vi "Write to DB_12202024.vi"(8 "error in (no error)":errorcluster, 11 "Database Entry in":refnum<class "Database Entry.lvclass">) -> (0 "error out":errorcluster, 2 "Stack names":string[](array[string]), 3 "Database Entry out":refnum<class "Database Entry.lvclass">)   [LabVIEW 2021, in "Database Entry.lvclass"]
uses:
  Database Entry.lvclass
  Database Entry.lvclass/Database Entry.ctl
  <vilib>/Utility/file.llb/Read Delimited Spreadsheet (string).vi
  <vilib>/Utility/file.llb/Write Delimited Spreadsheet (string).vi
  Components/Stack/Stack.lvclass
panel:
  out "Final name":string
  out "Data cluster":T1={"module or proto"="proto", " geometry"="full", "resolution"="LD", "baselayer"="BA_123", "toplayer"="SI_789", "bl_pos"="1", "tl_pos"="1", "put_pos"="1", "region"="1", "asstray"="1", "comptray"="1", "put"="1", "date"="2024-04-02", "timestart"="1:12:12.442", "timeend"="1:23:45.244", "operator"="cmuperson", "tape"="some", "glue"="some", "stack name"="some", "Adhesive type"="", "Comments"="", "Temperature"="", "Relative Humidity"=""}
  out "error out py":errorcluster
  out "String Out":string="Upload Success"
  in  "error in (no error) py":errorcluster
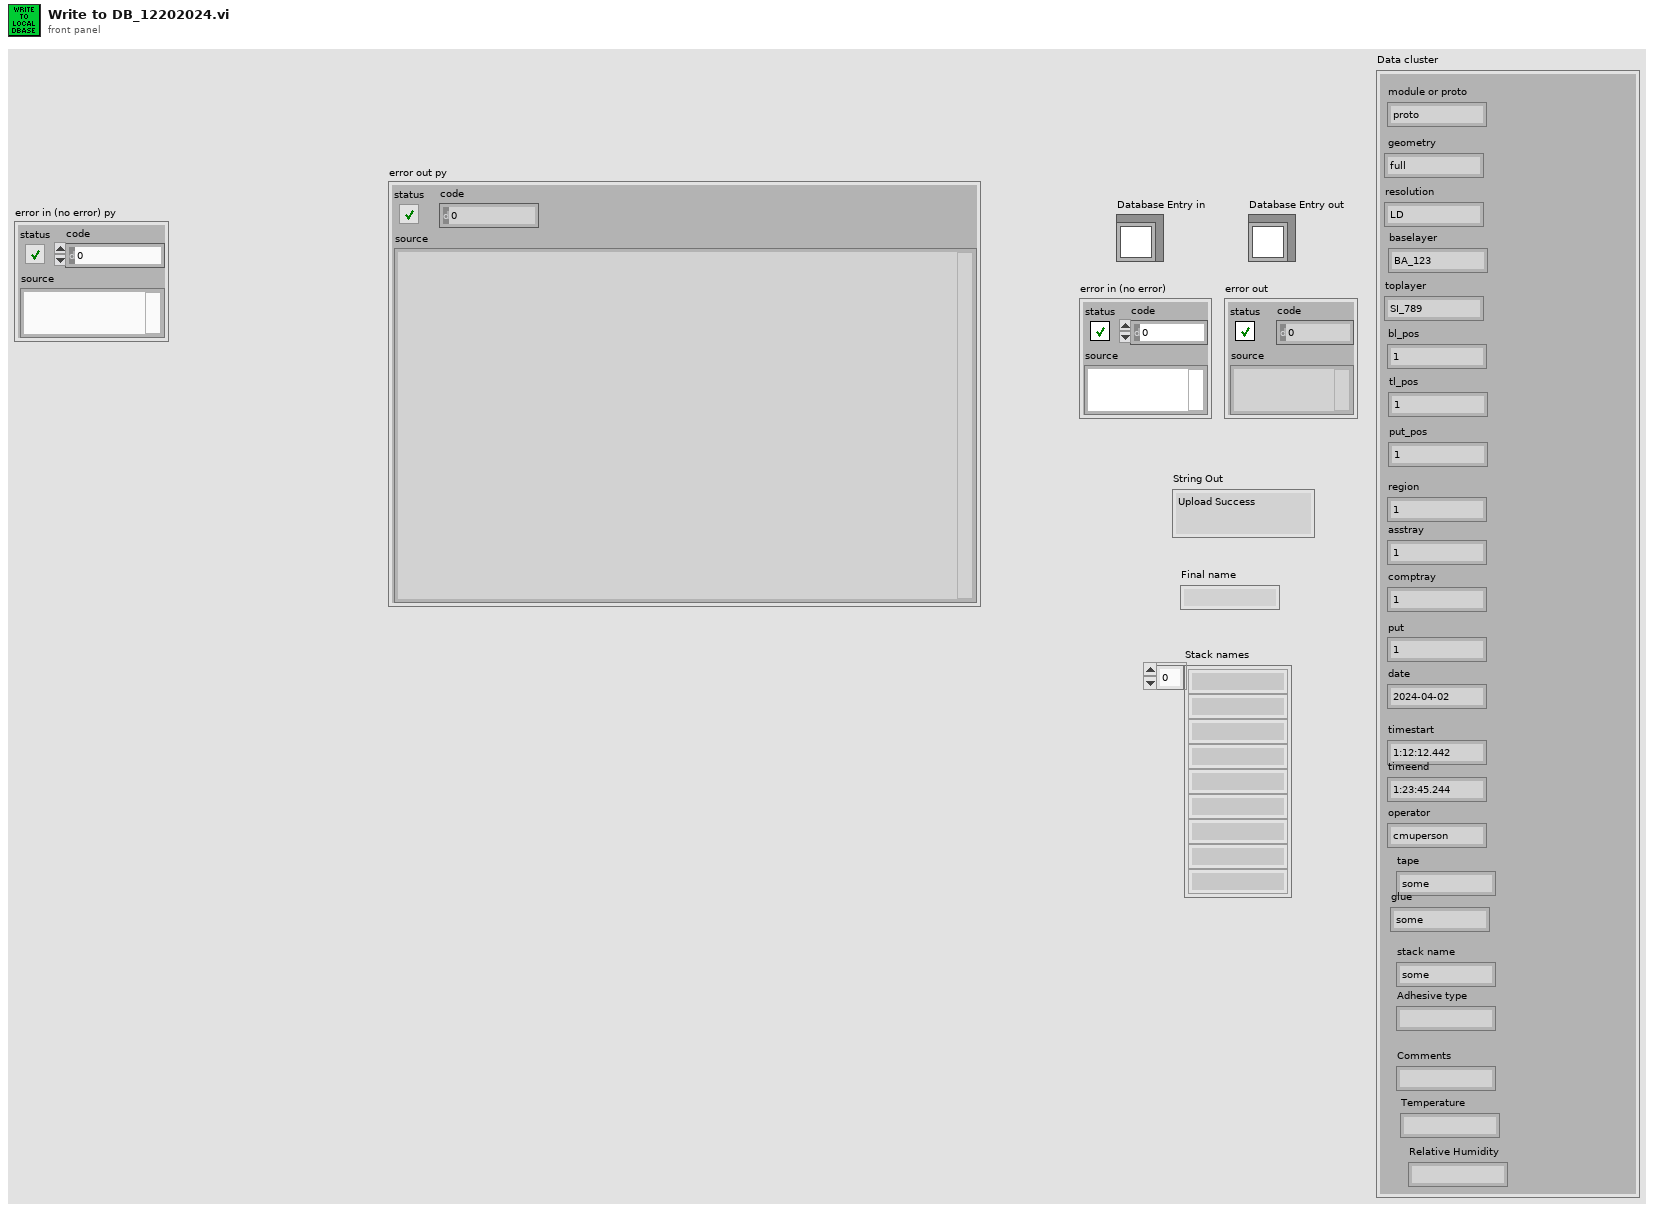
[diagram p1: front panel]
types:
  T1 = cluster{"module or proto":string, " geometry":string, "resolution":string, "baselayer":string, "toplayer":string, "bl_pos":string, "tl_pos":string, "put_pos":string, "region":string, "asstray":string, "comptray":string, "put":string, "date":string, "timestart":string, "timeend":string, "operator":string, "tape":string, "glue":string, "stack name":string, "Adhesive type":string, "Comments":string, "Temperature":string, "Relative Humidity":string}
  T2 = typedef "File Paths.ctl" = cluster{"Glue Pattern Folder":path, "Carrier Tray Folder":path, "Pick Up Tool Fixture Folder":path, "Components Folder":path, "Bellows Tool Offset.txt":path, "Pick Up Tool Offset.txt":path, "Dispense Tip Offset.txt":path, "Log Files":path, "Gantry Assembly Map.txt":path, "Syringe and offset map.txt":path, "Controllers Folder":path, "Local dbase config":path}
  T3 = cluster{"type":string, " geometry":string, "resolution":string, "baselayer":string, "toplayer":string, "bl_pos":string, "tl_pos":string, "put_pos":string, "region":string, "asstray":string, "comptray":string, "put":string, "date":string, "timestart":string, "timeend":string, "operator":string, "tape":string, "glue":string, "stack name":string, "Adhesive type":string, "Comments":string, "Temperature":string, "Relative Humidity":string}
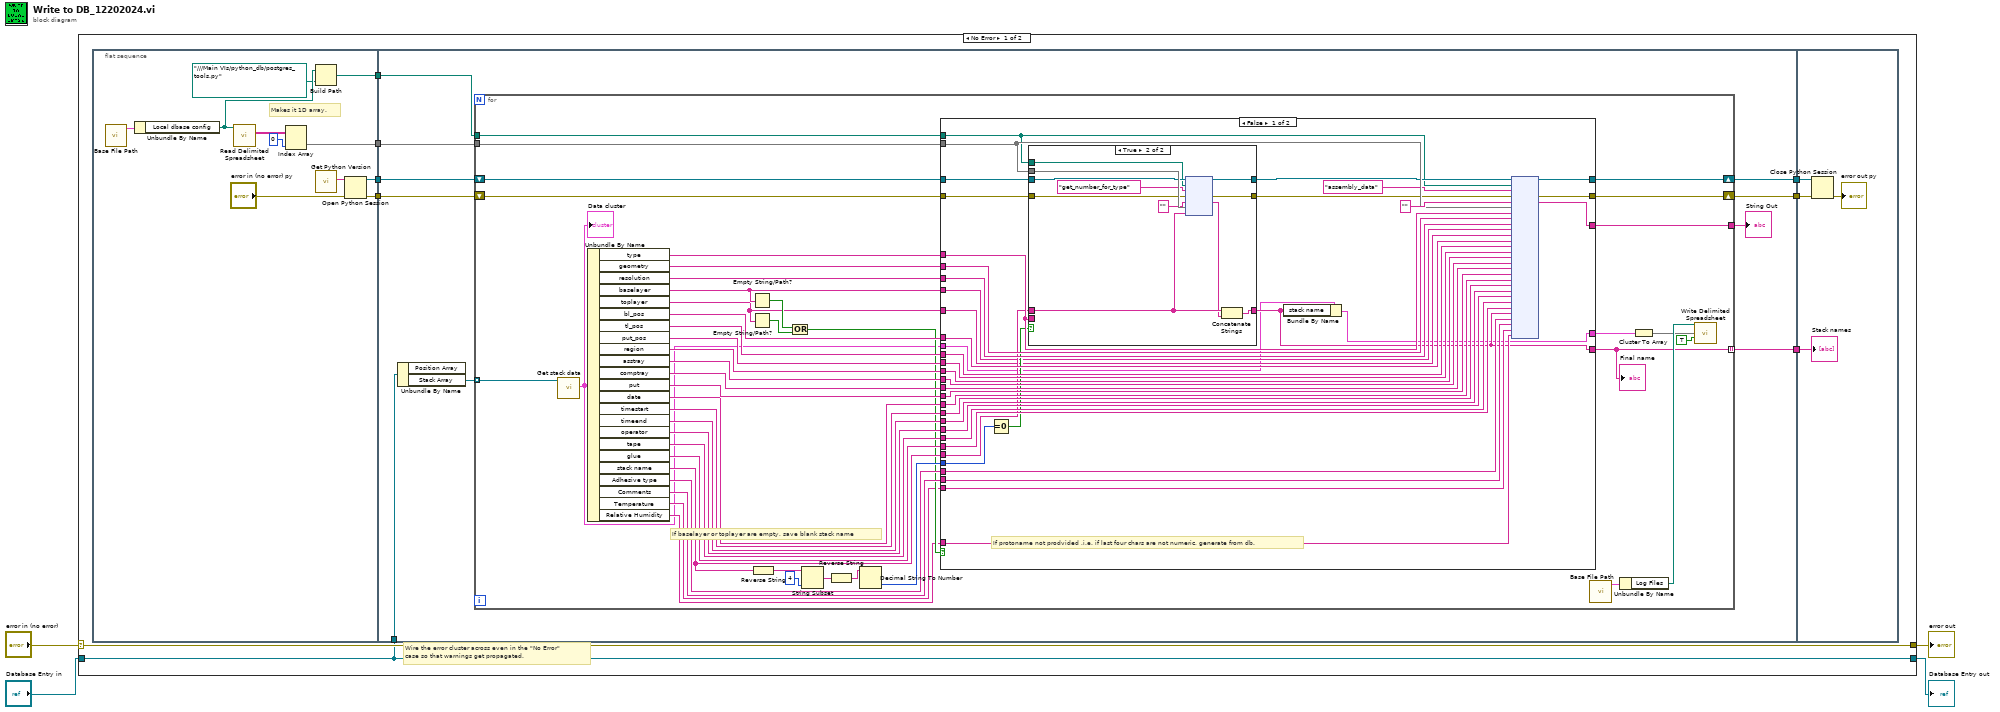
[diagram p0: block diagram]
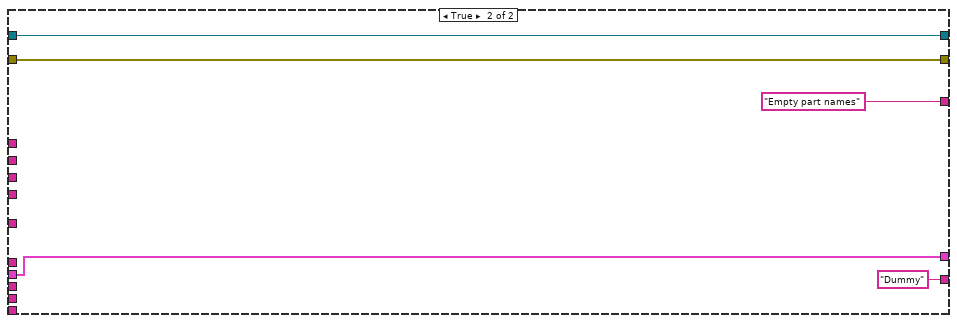
[diagram p3: hidden frame]
diagram:
  n1 = case shown="No Error" "error in (no error)" {
    selector: "error in (no error)" -> [w13 w144]
    tunnel: [w13 w144] -> w3
    tunnel: [w6 w143] -> w1
    tunnel: "Database Entry in" -> [w6 w143]
    frame No Error {
      # "Wire the error cluster across even in the \"No Error\"\ncase so that warnings get propagated."
      n2 = flat-sequence {
        tunnel: [w23] -> w12
        tunnel: [w24] -> w11
        tunnel: [w20] -> w10
        tunnel: [w16] -> w9
        tunnel: [w33] -> w8
        tunnel: [w32] -> w7
        tunnel: w12 -> [w34]
        tunnel: w11 -> [w31]
        tunnel: w10 -> [w30]
        tunnel: w9 -> [w29]
        tunnel: w6 -> [w28]
        tunnel: [w25] -> w5
        tunnel: w8 -> [w141]
        tunnel: w7 -> [w142]
        tunnel: w5 -> [w139]
        frame #0 {
          # "Makes it 1D array."
          n3 = call "Base File Path.vi"() -> ("Paths Out"=w21:T2)  [unwired: 11 in]
          n4 = Unbundle By Name(w21) -> ("Local dbase config"=w19:path)
          n5 = call-poly <vilib>:"Read Delimited Spreadsheet.vi"("file path (dialog if empty)"=w19) -> ("all rows"=w18:string[][])  [unwired: 9 in, 5 out]
          n6 = Index Array(array=w18, index (col)=0 ("disabled index (col)")) -> (element=w16:string[])  [unwired: 1 in]
          n7 = Build Path(base path=w19, name or relative path=path "../../../Main VIs/python_db/postgres_tools.py" ("module path")) -> (appended path=w20:path)
          n8 = call "Get Python Version.vi"() -> ("Python Version"=w14:string)  [unwired: 10 in, 1 out]
          n9 = Open Python Session(python version=w14, 3:"error in (no error) py") -> (session out=w24:refnum<k35>, error out=w23:errorcluster)  [unwired: 1 in]
        }
        frame #1 {
          n10 = Unbundle By Name(w28) -> ("Stack Array"=w26:refnum<class "Stack.lvclass">[])  [unwired: 1 out]
          n11 = for {
            tunnel: w30 -> [w57]
            shift-right: [w80] -> w33
            shift-left: w34 -> [w56]
            shift-right: [w79] -> w32
            shift-left: w31 -> [w58]
            tunnel: [w78] -> w27
            tunnel: w26 -> [w77] mode=indexing
            tunnel: w29 -> [w59]
            tunnel: [w42] -> w25 mode=indexing
            # "If baselayer or toplayer are empty, save blank stack name"
            n12 = call "Get stack data.vi"("Stack in"=w77) -> ("Data cluster"=w36:T3)  [unwired: 8 in, 2 out]
            "Data cluster" <- w36
            n13 = Unbundle By Name(w36) -> ("type"=w60:string, "geometry"=w76:string, "resolution"=w75:string, "baselayer"=w46:string, "toplayer"=w44:string, "bl_pos"=w74:string, "tl_pos"=w73:string, "put_pos"=w72:string, "region"=w55:string, "asstray"=w71:string, "comptray"=w70:string, "put"=w69:string, "date"=w68:string, "timestart"=w67:string, "timeend"=w66:string, "operator"=w65:string, "tape"=w64:string, "glue"=w63:string, "stack name"=w47:string, "Adhesive type"=w54:string, "Comments"=w53:string, "Temperature"=w40:string, "Relative Humidity"=w39:string)
            n14 = Empty String/Path?(string/path=w46) -> (empty?=w45:bool)
            n15 = Empty String/Path?(string/path=w44) -> (empty?=w43:bool)
            n16 = Reverse String(1:w47) -> (0:w52:string)
            n17 = Or(x=w45, y=w43) -> (x .or. y?=w41:bool)
            n18 = String Subset(string=w52, length (rest)=4 ("length (rest)")) -> (substring=w50:string)  [unwired: 1 in]
            n19 = Reverse String(1:w50) -> (0:w49:string)
            n20 = Decimal String To Number(string=w49) -> (number=w48:i32)  [unwired: 2 in, 1 out]
            n21 = case shown="False" w41 {
              tunnel: [w119 w137] -> w80
              tunnel: [w118 w138] -> w79
              tunnel: [w117 "Empty part names"] -> w78
              tunnel: w76 -> [w115 _]
              tunnel: w75 -> [w114 _]
              tunnel: w74 -> [w113 _]
              tunnel: w73 -> [w112 _]
              tunnel: w72 -> [w111 _]
              tunnel: w71 -> [w110 _]
              tunnel: w70 -> [w109 _]
              tunnel: w69 -> [w108 _]
              tunnel: w68 -> [w107 _]
              tunnel: w67 -> [w106 _]
              tunnel: w66 -> [w105 _]
              tunnel: w65 -> [w104 _]
              tunnel: w64 -> [w103 _]
              tunnel: w63 -> [w102 _]
              tunnel: w60 -> [w101 _]
              tunnel: w59 -> [w100 _]
              tunnel: w58 -> [w99 w138]
              tunnel: w57 -> [w97 _]
              tunnel: w56 -> [w96 w137]
              tunnel: w55 -> [w93 _]
              tunnel: w54 -> [w92 _]
              tunnel: w53 -> [w91 _]
              tunnel: w48 -> [w90 _]
              tunnel: w47 -> [w89 _]
              tunnel: w46 -> [w87 _]
              tunnel: w44 -> [w86 _]
              tunnel: [w83 "Dummy" ("stack name")] -> w42
              tunnel: w40 -> [w85 _]
              tunnel: w39 -> [w84 _]
              tunnel: w36 -> [w82 w134]
              tunnel: [w81 w134] -> w35
              frame False {
                # "If protoname not prodvided ,i.e. if last four chars are not numeric, generate from db."
                n22 = Equal To 0?(x=w90) -> (x = 0?=w88:bool)
                n23 = case shown="True" w88 {
                  tunnel: w101 -> [_ _]
                  tunnel: w89 -> [w120 w133]
                  tunnel: w100 -> [_ w132]
                  tunnel: w99 -> [w122 w131]
                  tunnel: [w122 w130] -> w98
                  tunnel: w97 -> [_ w129]
                  tunnel: w96 -> [w121 w128]
                  tunnel: [w121 w127] -> w95
                  tunnel: [w120 w126] -> w83
                  frame False {
                  }
                  frame True {
                    n24 = node(w131, w129, "get_number_for_type" ("function name"), w128, "" ("function name"), w132, w133) -> (w130:refnum<k35>, w127:errorcluster, w123:string)  [unwired: 2 in, 2 out]
                    n25 = Concatenate Strings(w133, w123) -> (w126:string)
                  }
                }
                n26 = Bundle By Name(cluster=w82, "stack name"=w83) -> (w81:T3)
                n27 = node(w98, w97, "assembly_data" ("function name"), w95, "", w100, w101, w115, w114, w87, w86, w113, w112, w111, w93, w110, w109, w108, w107, w106, w105, w104, w103, w102, w83, w92, w91, w85, w84) -> (w118:refnum<k35>, w119:errorcluster, w117:string)  [unwired: 24 in, 2 out]
              }
              frame True {
              }
            }
            "Final name" <- w42
            n28 = call "Base File Path.vi"() -> ("Paths Out"=w62:T2)  [unwired: 11 in]
            n29 = Unbundle By Name(w62) -> ("Log Files"=w61:path)
            n30 = Cluster To Array(cluster=w35) -> (array=w37:string[])
            n31 = call-poly <vilib>:"Write Delimited Spreadsheet.vi"("file path (dialog if empty)"=w61, "1D data"=w37, "append to file? (new file:F)"=TRUE) -> ()  [unwired: 11 in, 2 out]
          }
          "String Out" <- w27
        }
        frame #2 {
          n32 = Close Python Session(session in=w142, error in=w141) -> (11:→"error out py":errorcluster)
          "Stack names" <- w139
        }
      }
    }
    frame Error {
    }
  }
  "error out" <- w3
  "Database Entry out" <- w1
